vi "Rename VI.vi"(5 "Project":refnum<vi>, 8 "error in":errorcluster, 9 "new vi name":string, 10 "vi path":path, 11 "Application":refnum<vi>) -> (0 "error out":errorcluster, 3 "dup Application":refnum<vi>)   [LabVIEW 2013, in "TagBusProcessingPluginFeatureDecider.lvclass"]
uses:
  TagBusProcessingPluginFeatureDecider.lvclass
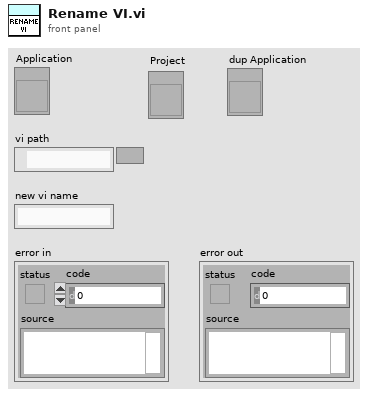
[diagram p1: front panel]
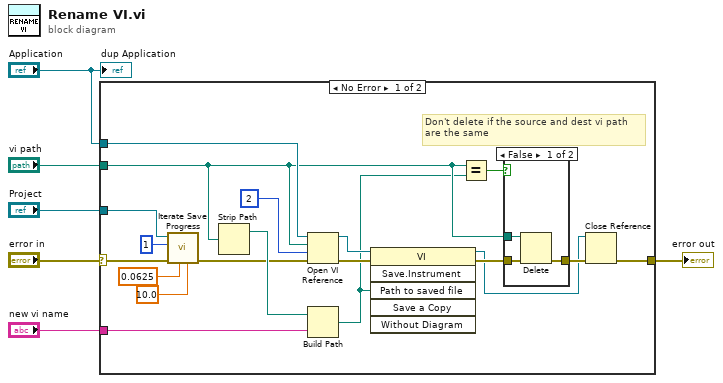
[diagram p0: block diagram]
diagram:
  n1 = case shown="No Error" "error in" {
    selector: "error in" -> [w9 w30]
    tunnel: "Application" -> [w25 _]
    tunnel: "new vi name" -> [w22 _]
    tunnel: [w18 w30] -> w4
    tunnel: "vi path" -> [w15 _]
    tunnel: "Project" -> [w7 _]
    frame No Error {
      # "Don't delete if the source and dest vi path\nare the same"
      n2 = call <resource>:"Iterate Save Progress.vi"("Total Iteration Progress"=10.0 ("This Task's Percentage"), "This Task's Percentage"=0.0625, "error in (no error)"=w9, "Total Iterations (this task)"=1, "Project"=w7) -> ("error out"=w8:errorcluster)  [unwired: 6 in]
      n3 = Strip Path(path=w15) -> (stripped path=w23:path)  [unwired: 1 out]
      n4 = Open VI Reference(application reference (local)=w25, vi path=w15, options=2 ("Template VIs as templates"), error in (no error)=w8) -> (vi reference=w24:refnum<vi>, error out=w20:errorcluster)  [unwired: 2 in]
      n5 = Build Path(base path=w23, name or relative path=w22) -> (appended path=w13:path)
      n6 = invoke class="VI" method="Save.Instrument"(reference=w24, error in=w20, "Path to saved file"=w13) -> (reference out=w17:refnum<vi>, error out=w21:errorcluster)  [unwired: 3 in, 4 out]
      n7 = Equal?(x=w15, y=w13) -> (x = y?=w14:bool)
      n8 = case shown="False" w14 {
        tunnel: w15 -> [w28 _]
        tunnel: w21 -> [w27 w29]
        tunnel: [w26 w29] -> w19
        frame False {
          n9 = Delete(path (use dialog)=w28, error in=w27) -> (error out=w26:errorcluster)  [unwired: 3 in, 2 out]
        }
        frame True {
        }
      }
      n10 = Close Reference(reference=w17, error in (no error)=w19) -> (error out=w18:errorcluster)
    }
    frame Error {
    }
  }
  "error out" <- w4
  "dup Application" <- "Application"
